vi "4.6.1.vi"() -> ()   [LabVIEW 2017]
panel:
  in  "停止":bool
  out "x+y":dbl
  in  "数值 2":dbl
  in  "数值":dbl
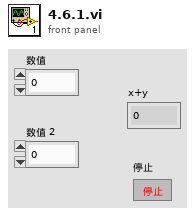
[diagram p1: front panel]
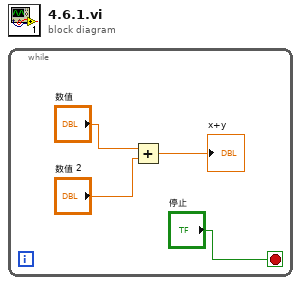
[diagram p0: block diagram]
diagram:
  n1 = while {
    stop <- "停止" stop-if-true
    n2 = Add(x="数值", y="数值 2") -> (x+y=→"x+y":dbl)
  }
